vi "Test ColorSelector.vi"() -> ()   [LabVIEW 2015, in "ColorSelector.lvclass"]
doc: "This VI tests all the functions of the <b>ColorSelector QControl</b>. It is also an example of how to implement using this QControl. However, normal use <b>does not require</b> that the VI using this QControl be part of the <b>ColorSelector QControl Class</b>.\n<b> </b> <b> </b>\n©2017 Q Software Innovations, LLC (QSI)\nwritten by Quentin Alldredge\nproduced in LabVIEW 2015\n\nsupport@qsoftwareinnovations.com\nwww.qsoftwareinnovations.com\n\nAll rights reserved.\n\nRedistribution and use in source and binary forms, with or without modification, are permitted provided that the following conditions are met:\n\n * Redistributions of source code must retain the above copyright notice, this list of conditions and the following disclaimer.\n * Redistributions in binary form must reproduce the above copyright notice, this list of conditions and the following disclaimer in the documentation and/or other materials provided with the distribution.\n * Neither the name of Q Software Innovations, LLC. nor the names of its contributors may be used to endorse or promote products derived from this software without specific prior written permission.\n\nTHIS SOFTWARE IS PROVIDED BY THE COPYRIGHT HOLDERS AND CONTRIBUTORS \"AS IS\" AND ANY EXPRESS OR IMPLIED WARRANTIES, INCLUDING, BUT NOT LIMITED TO, THE IMPLIED WARRANTIES OF MERCHANTABILITY AND FITNESS FOR A PARTICULAR PURPOSE ARE DISCLAIMED. IN NO EVENT SHALL THE COPYRIGHT OWNER OR CONTRIBUTORS BE LIABLE FOR ANY DIRECT, INDIRECT, INCIDENTAL, SPECIAL, EXEMPLARY, OR CONSEQUENTIAL DAMAGES (INCLUDING, BUT NOT LIMITED TO, PROCUREMENT OF SUBSTITUTE GOODS OR SERVICES; LOSS OF USE, DATA, OR PROFITS; OR BUSINESS INTERRUPTION) HOWEVER CAUSED AND ON ANY THEORY OF LIABILITY, WHETHER IN CONTRACT, STRICT LIABILITY, OR TORT (INCLUDING NEGLIGENCE OR OTHERWISE) ARISING IN ANY WAY OUT OF THE USE OF THIS SOFTWARE, EVEN IF ADVISED OF THE POSSIBILITY OF SUCH DAMAGE."
uses:
  ColorSelector.lvclass
  Color Selector Facade.ctl
  Named Colors Enum.ctl
  Write Set Selected Color.vi
panel:
  out "RYB Compementary Color":u32(colorbox)
  out "RGB Compementary Color":u32(colorbox)
  in  "K (%)":dbl format="%#.0f"
  in  "M (%)":dbl format="%#.0f"
  in  "Y (%)":dbl format="%#.0f"
  in  "C (%)":dbl format="%#.0f"
  in  "S (%)":dbl format="%#.0f"
  in  "L (%)":dbl format="%#.1f"
  in  "H (°)":dbl format="%#.0f"
  in  "Named Colors":T1
  in  "Set Color":u32(colorbox)
  in  "Color Selector QControl":T2 {"Hex Representation" format="%06x"}
  # "Test Inputs"
  # "Other Information"
  # "Other Color Scales"
  # "HSL"
  # "CMYK"
  # "°  = 0-360"
  # "% = 0-100"
  # "RGB"
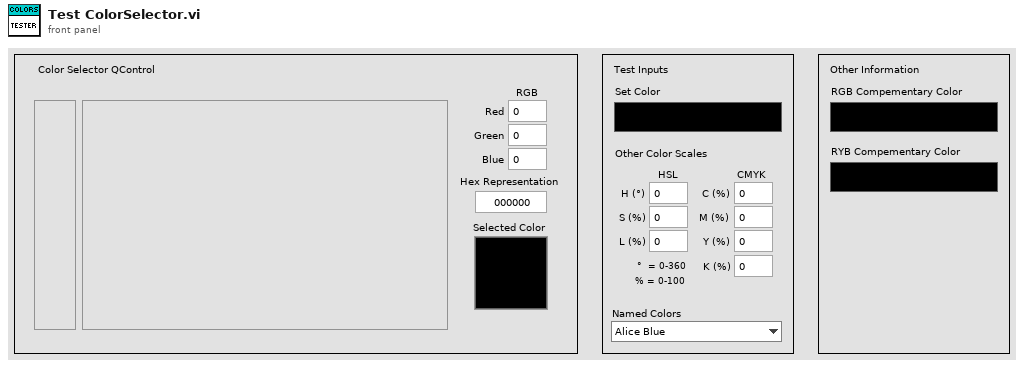
[diagram p1: front panel]
types:
  T1 = typedef "ColorSelector.lvclass/Named Colors Enum.ctl" = enum16{"Alice Blue", "Antique White", "Aqua Marine", "Azure", "Beige", "Bisque", "Black", "Blanched Almond", "Blue", "Blue Violet", "Brown", "Burly Wood", "Cadet Blue", "Chart Reuse", "Chocolate", "Coral", "Corn Flower Blue", "Corn Silk", "Crimson", "Cyan / Aqua", "Dark Blue", "Dark Cyan", "Dark Golden Rod", "Dark Gray / Dark Grey", "Dark Green", "Dark Khaki", "Dark Magenta", "Dark Olive Green", "Dark Orange", "Dark Orchid", "Dark Red", "Dark Salmon", "Dark Sea Green", "Dark Slate Blue", "Dark Slate Gray", "Dark Turquoise", "Dark Violet", "Deep Pink", "Deep Sky Blue", "Dim Gray / Dim Grey", "Dodger Blue", "Firebrick", "Floral White", "Forest Green", "Gainsboro", "Ghost White", "Gold", "Golden Rod", "Gray / Grey", "Green", "Green Yellow", "Honeydew", "Hot Pink", "Indian Red", "Indigo", "Ivory", "Khaki", "Lavender", "Lavender Blush", "Lawn Green", "Lemon Chiffon", "Light Blue", "Light Coral", "Light Cyan", "Light Golden Rod Yellow", "Light Gray / Light Grey", "Light Green", "Light Pink", "Light Salmon", "Light Sea Green", "Light Sky Blue", "Light Slate Gray", "Light Steel Blue", "Light Yellow", "Lime", "Lime Green", "Linen", "Magenta / Fuchsia", "Maroon", "Medium Aqua Marine", "Medium Blue", "Medium Orchid", "Medium Purple", "Medium Sea Green", "Medium Slate Blue", "Medium Spring Green", "Medium Turquoise", "Medium Violet Red", "Midnight Blue", "Mint Cream", "Misty Rose", "Moccasin", "Navajo White", "Navy", "Old Lace", "Olive", "Olive Drab", "Orange", "Orange Red", "Orchid", "Pale Golden Rod", "Pale Green", "Pale Turquoise", "Pale Violet Red", "Papaya Whip", "Peach Puff", "Peru", "Pink", "Plum", "Powder Blue", "Purple", "RYB Primary Blue", "RYB Primary Red", "RYB Primary Yellow", "RYB Secondary Green", "RYB Secondary Orange", "RYB Secondary Purple", "RYB Tertiary Amber", "RYB Tertiary Chartreuse", "RYB Tertiary Magenta", "RYB Tertiary Teal", "RYB Tertiary Vermillion", "RYB Tertiary Violet", "Red", "Rosy Brown", "Royal Blue", "Saddle Brown", "Salmon", "Sandy Brown", "Sea Green", "Sea Shell", "Sienna", "Silver", "Sky Blue", "Slate Blue", "Slate Gray", "Snow", "Spring Green", "Steel Blue", "Tan", "Teal", "Thistle", "Tomato", "Turquoise", "Violet", "Wheat", "White", "White Smoke", "Yellow", "Yellow Green"}
  T2 = typedef "ColorSelector.lvclass/Color Selector Facade.ctl" = cluster{"Grey Selector":picture, "Color Selector":picture, "Red":u8, "Green":u8, "Blue":u8, "Hex Representation":u32, "Selected Color":u32}
  T3 = typedef "lveventtype.ctl" = enum32{"Null", "Timeout", "Annotation Menu Selection", "Annotation Menu Selection?", "App Instance Close", "App Instance Close?", "Autoscale Range Change", "Bookmark Info Change", "Cell Edit", "Cell Edit?", "Cursor Grab", "Cursor Grab?", "Cursor Menu Selection", "Cursor Menu Selection?", "Cursor Move", "Cursor Release", "Data Change", "Direction Change", "Display State Change", "Drag Ended", "Drag Enter", "Drag Leave", "Drag Over", "Drag Source Update", "Drag Starting", "Drag Starting?", "Drop", "Exec State Change", "Key Down", "Key Down?", "Key Repeat", "Key Repeat?", "Key Up", "Listbox Double Click", "Menu Activation?", "Menu Selection (App)", "Menu Selection? (App)", "Menu Selection (User)", "Mouse Down", "Mouse Down?", "Mouse Enter", "Mouse Leave", "Mouse Move", "Mouse Up", "Mouse Wheel", "NI Security User Change (App)", "Pane Size", "Panel Close", "Panel Close?", "Panel Resize", "Plot Attribute Change", "Scale Range Change", "Shortcut Menu Activation?", "Shortcut Menu Selection (App)", "Shortcut Menu Selection? (App)", "Shortcut Menu Selection (User)", "Tree Double Click", "Tree Drag", "Tree Drag?", "Tree Drop", "Tree Drop?", "Tree Item Close", "Tree Item Close?", "Tree Item Open", "Tree Item Open?", "User Event", "Value Change"}
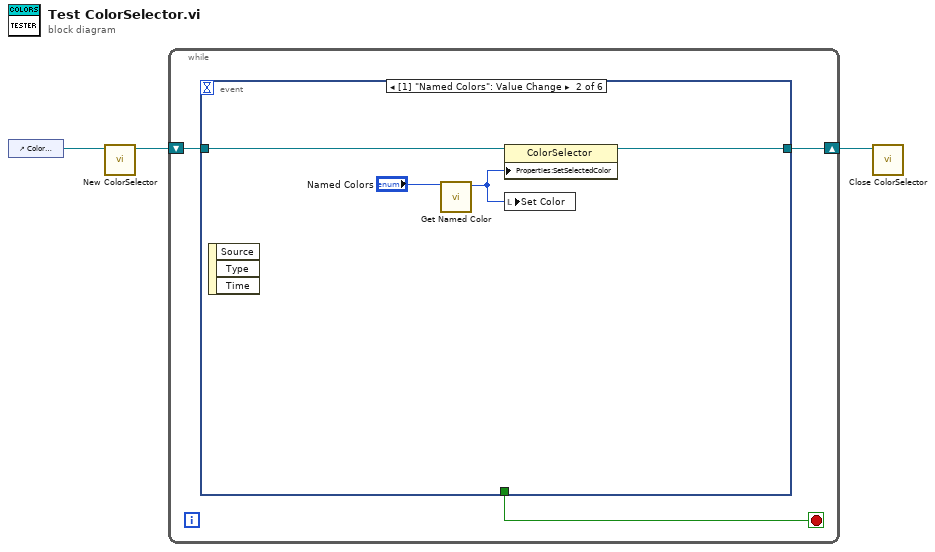
[diagram p0: block diagram]
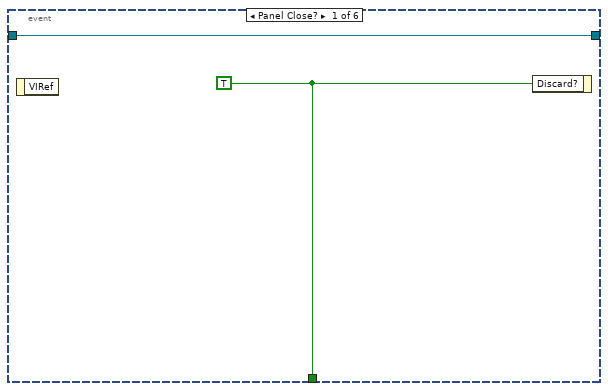
[diagram p2: hidden frame]
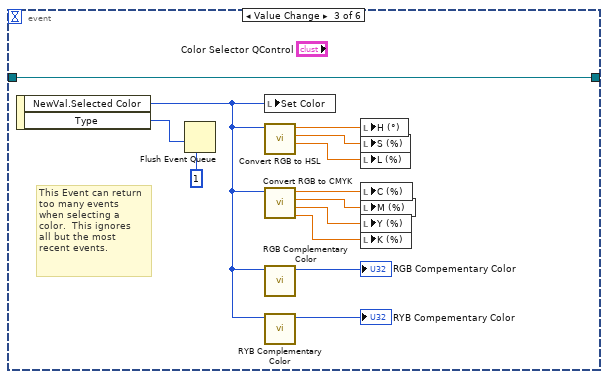
[diagram p3: hidden frame]
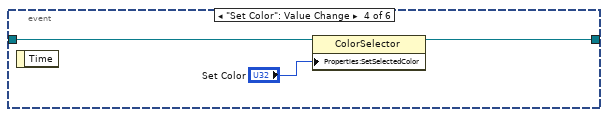
[diagram p4: hidden frame]
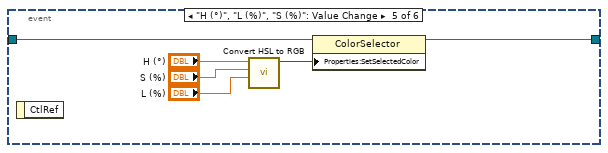
[diagram p5: hidden frame]
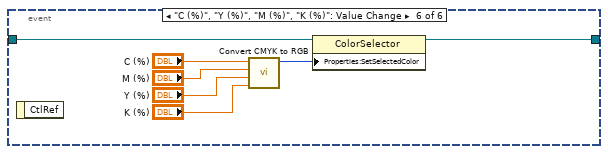
[diagram p6: hidden frame]
diagram:
  n1 = control-ref of="Color Selector QControl"() -> (w3:refnum<vi>)
  n2 = call "New ColorSelector.vi"("Reference"=w3) -> ("ColorSelector out"=w2:refnum<class "ColorSelector.lvclass">)  [unwired: 9 in, 1 out]
  n3 = while {
    shift-right: [w4] -> w1
    shift-left: w2 -> [w5]
    stop <- w6 stop-if-true
    n4 = event shown="[1] \"Named Colors\": Value Change" {
      selector: _ -> [_ _ _ _ _ _]
      dyn-events: _ -> [_ _ _ _ _ _]
      timeout: _ -> [_ _ _ _ _ _]
      tunnel: [w8 _ _ _ _ _] -> w6
      tunnel: w5 -> [w7 w12 w25 w28 w31 w37]
      tunnel: [w7 w11 w25 w27 w30 w36] -> w4
      event Panel Close? {
        w8 = TRUE ("Discard?")
        n5 = event-data() -> ()  [unwired: 1 in, 1 out]
        n6 = event-data("Discard?"=w8) -> ()  [unwired: 1 in, 1 out]
      }
      event Value Change {
        n7 = event-data() -> ()  [unwired: 1 in, 3 out]
        n8 = call "Get Named Color.vi"("Named Colors"="Named Colors") -> ("Color out"=w9:u32)  [unwired: 9 in, 1 out]
        n9 = property class="ColorSelector"(reference=w12, "Properties:SetSelectedColor"=w9) -> (reference out=w11:refnum<class "ColorSelector.lvclass">)  [unwired: 1 in, 1 out]
        n10 = local write "Set Color"(w9) -> ()
      }
      event Value Change {
        # "This Event can return\ntoo many events\nwhen selecting a \ncolor.  This ignores \nall but the most\nrecent events."
        n11 = event-data() -> ("NewVal.Selected Color"=w16:u32, "Type"=w14:T3)  [unwired: 1 in]
        n12 = Flush Event Queue(2:w14, 5:1 ("keep most recent")) -> ()  [unwired: 4 in, 3 out]
        n13 = local write "Set Color"(w16) -> ()
        n14 = call "Convert RGB to HSL.vi"("Color Box"=w16) -> ("L (%)"=w22:dbl, "S (%)"=w23:dbl, "H (deg)"=w24:dbl)  [unwired: 8 in]
        n15 = call "Convert RGB to CMYK.vi"("Color in"=w16) -> ("K (%)"=w18:dbl, "Y (%)"=w19:dbl, "M (%)"=w20:dbl, "C (%)"=w21:dbl)  [unwired: 7 in]
        n16 = call "RGB Complementary Color.vi"("Color in"=w16) -> ("Complementary Color"=→"RGB Compementary Color":u32)  [unwired: 10 in]
        n17 = call "RYB Complementary Color.vi"("Color in"=w16) -> ("Complementary Color"=→"RYB Compementary Color":u32)  [unwired: 10 in]
        n18 = local write "H (°)"(w24) -> ()
        n19 = local write "S (%)"(w23) -> ()
        n20 = local write "L (%)"(w22) -> ()
        n21 = local write "C (%)"(w21) -> ()
        n22 = local write "M (%)"(w20) -> ()
        n23 = local write "Y (%)"(w19) -> ()
        n24 = local write "K (%)"(w18) -> ()
      }
      event "Set Color": Value Change {
        n25 = event-data() -> ()  [unwired: 1 in, 1 out]
        n26 = property class="ColorSelector"(reference=w28, "Properties:SetSelectedColor"="Set Color") -> (reference out=w27:refnum<class "ColorSelector.lvclass">)  [unwired: 1 in, 1 out]
      }
      event "H (°)", "L (%)", "S (%)": Value Change {
        n27 = event-data() -> ()  [unwired: 1 in, 1 out]
        n28 = call "Convert HSL to RGB.vi"("L (%)"="L (%)", "S (%)"="S (%)", "H (deg)"="H (°)") -> ("Color Box"=w29:u32)  [unwired: 8 in]
        n29 = property class="ColorSelector"(reference=w31, "Properties:SetSelectedColor"=w29) -> (reference out=w30:refnum<class "ColorSelector.lvclass">)  [unwired: 1 in, 1 out]
      }
      event "C (%)", "Y (%)", "M (%)", "K (%)": Value Change {
        n30 = event-data() -> ()  [unwired: 1 in, 1 out]
        n31 = call "Convert CMYK to RGB.vi"("K (%)"="K (%)", "Y (%)"="Y (%)", "M (%)"="M (%)", "C (%)"="C (%)") -> ("Color out"=w35:u32)  [unwired: 7 in]
        n32 = property class="ColorSelector"(reference=w37, "Properties:SetSelectedColor"=w35) -> (reference out=w36:refnum<class "ColorSelector.lvclass">)  [unwired: 1 in, 1 out]
      }
    }
  }
  n33 = call "Close ColorSelector.vi"("ColorSelector in"=w1) -> ()  [unwired: 10 in, 1 out]
